vi "Configure Band.vi"(6 "Variable High Frequency Filter (0)":dbl, 7 "High Frequency Filter (0: adFsdiv2)":i32(ring) items=["adFsdiv2", "adHzVar", "adHzAES20k", "adHzAES40k", "adHzAES80k"], 8 "error in (no error)":errorcluster, 9 "Low Frequency Filter (0: adDC)":i32(ring) items=["adDC", "adHz22", "adHz100", "adHz400", "adSharp400", "adHzAES20", "adHzAES40", "adHzES80"], 10 "Analyzer (0: A0)":i32(ring) items=["A0", "A1"], 11 "VISA resource name":refnum<visa-resource-name>) -> (0 "error out":errorcluster, 3 "VISA resource name out":refnum<visa-resource-name>)   [LabVIEW 2014, in "Stanford Research SR1.lvlib"]
doc: "Configures the attributes for the Band."
uses:
  Stanford Research SR1.lvlib
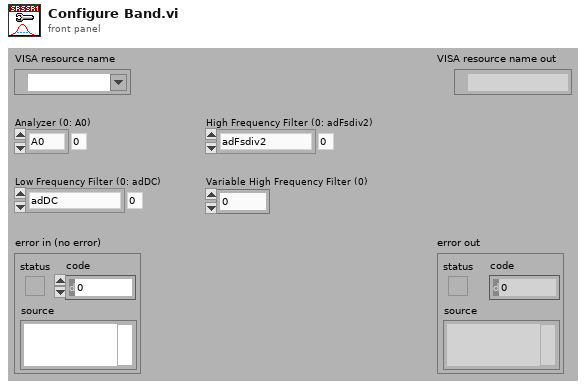
[diagram p1: front panel]
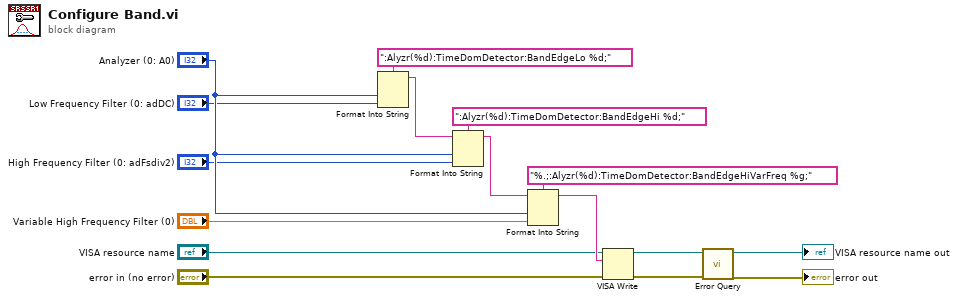
[diagram p0: block diagram]
diagram:
  n1 = Format Into String(format string=":Alyzr(%d):TimeDomDetector:BandEdgeLo %d;", "Analyzer (0: A0)", "Low Frequency Filter (0: adDC)") -> (resulting string=w15:string)  [unwired: 2 in, 1 out]
  n2 = Format Into String(format string=":Alyzr(%d):TimeDomDetector:BandEdgeHi %d;", initial string=w15, "Analyzer (0: A0)", "High Frequency Filter (0: adFsdiv2)") -> (resulting string=w13:string)  [unwired: 1 in, 1 out]
  n3 = Format Into String(format string="%.;:Alyzr(%d):TimeDomDetector:BandEdgeHiVarFreq %g;", initial string=w13, "Analyzer (0: A0)", "Variable High Frequency Filter (0)") -> (resulting string=w11:string)  [unwired: 1 in, 1 out]
  n4 = VISA Write(VISA resource name="VISA resource name", write buffer=w11, error in (no error)="error in (no error)") -> (VISA resource name out=w8:refnum<visa-resource-name>, error out=w7:errorcluster)  [unwired: 1 out]
  n5 = call "Error Query.vi"("error in (no error)"=w7, "VISA resource name"=w8) -> ("error out"=→"error out":errorcluster, "VISA resource name out"=→"VISA resource name out":refnum<visa-resource-name>)  [unwired: 6 in, 2 out]
